vi "Global 1.vi"() -> ()   [LabVIEW 2016]
panel:
  in  "stop 2":bool
  in  "stop":bool
  in  "Boolean 2":bool
  in  "Boolean":bool
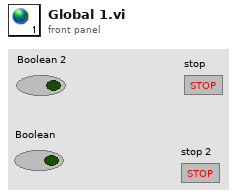
[diagram p1: front panel]
diagram:
